vi "SeCrTS-DD Queue Data log module.vi"(8 "error in":errorcluster) -> (0 "error out":errorcluster)   [LabVIEW 2022 SP3]
uses:
  Control/SeCrTS-Datalog enumDD.ctl
  Globals/SeCrTS-DD globals.vi
panel:
  out "x":u32
  out "x-y":dbl
  out "Restart":bool
  out "Log health":bool=TRUE
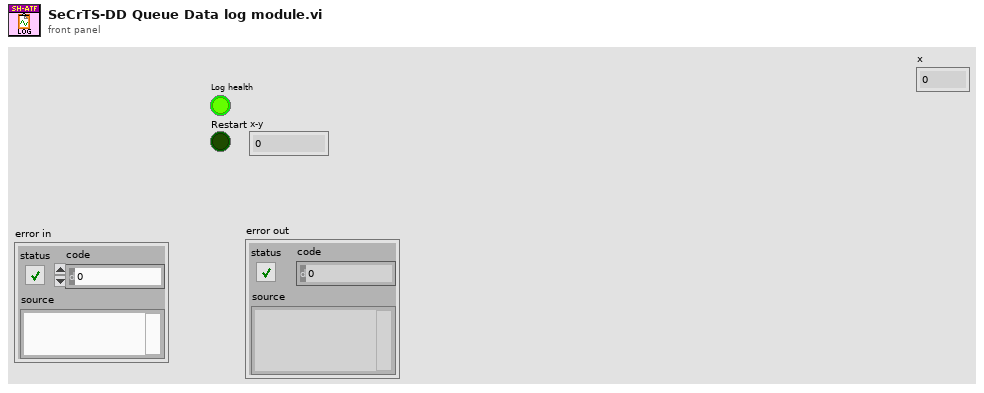
[diagram p1: front panel]
types:
  T1 = cluster{"Log In Progress?":bool, "Log Start Time":timestamp, "Analog Queues":refnum<queue>[], "Digital Queues":refnum<queue>[], "tdms file ref":refnum<k34>}
  T2 = typedef "SeCrTS-Datalog enumDD.ctl" = enum16{"Initialize", "Poll", "Create file", "log Analog", "log Digital", "Flush Queues", "Close file", "Error", "Exit"}
  T3 = enum16{"open", "open or create", "create or replace", "create", "open (read-only)"}
  T4 = cluster{"Datalog path":path, "Configuration path":path, "Signal list path":path, "Sub vi's":path, "Authentication":path}
  T5 = cluster{"Channel names":cluster{"AI_C_Data P":string[], "AI_V_Data P":string[], "AO_Data P":string[], "DO_Data P":string[], "ACC_Data P":string[], "TC Data P":string[], "Drive_A_C":string[], "Drive_A_D":string[], "AI_C_Data S":string[], "DO_Data S":string[]}, "DI Names":cluster{"Di P":string[], "Di S":string[]}}
  T6 = cluster{"AI_C_Data P":string[], "AI_V_Data P":string[], "AO_Data P":string[], "DO_Data P":string[], "ACC_Data P":string[], "TC Data P":string[], "Drive_A_C":string[], "Drive_A_D":string[], "AI_C_Data S":string[], "DO_Data S":string[]}
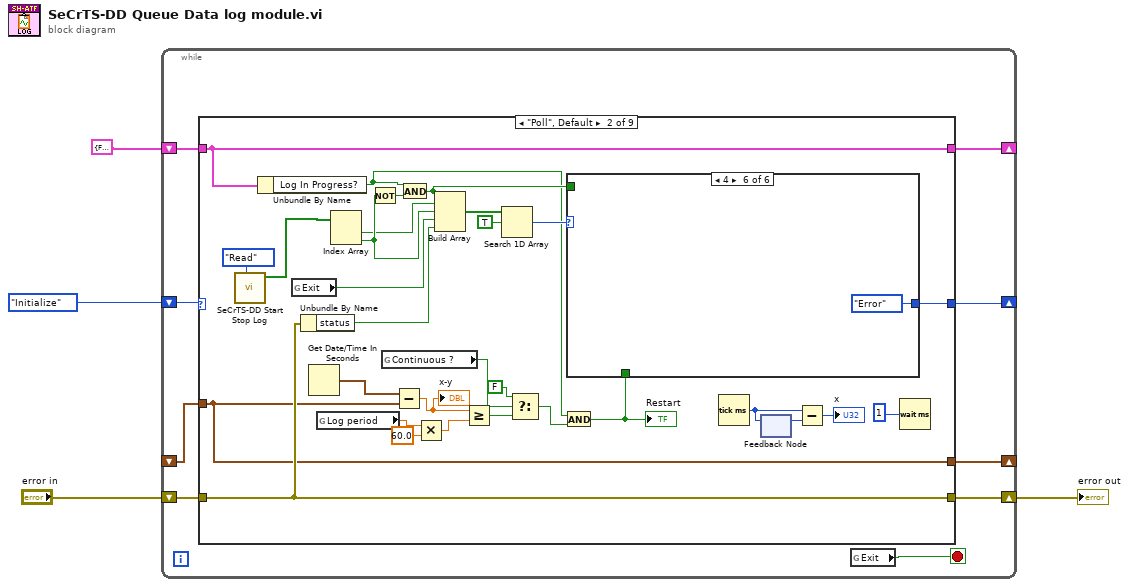
[diagram p0: block diagram]
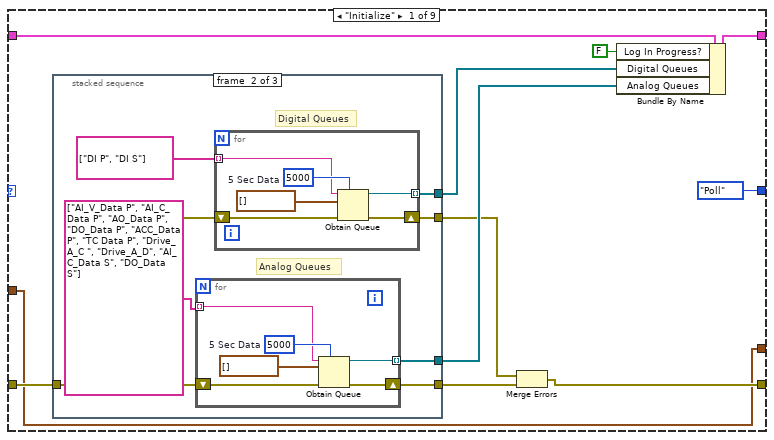
[diagram p2: hidden frame]
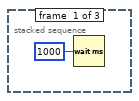
[diagram p3: hidden frame]
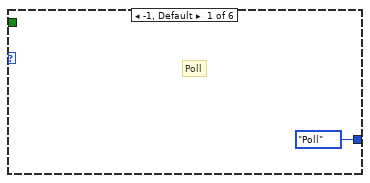
[diagram p5: hidden frame]
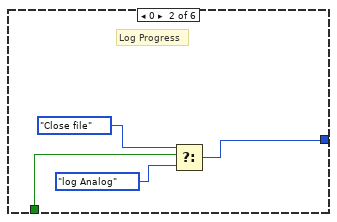
[diagram p6: hidden frame]
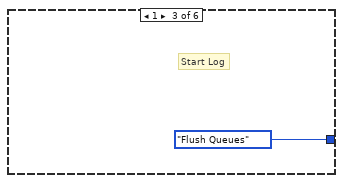
[diagram p7: hidden frame]
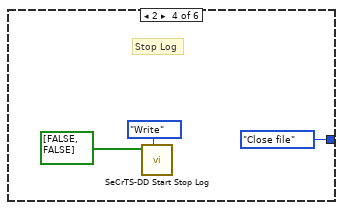
[diagram p8: hidden frame]
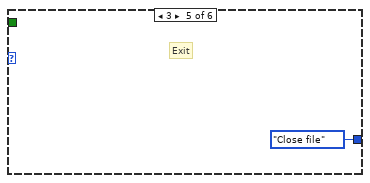
[diagram p9: hidden frame]
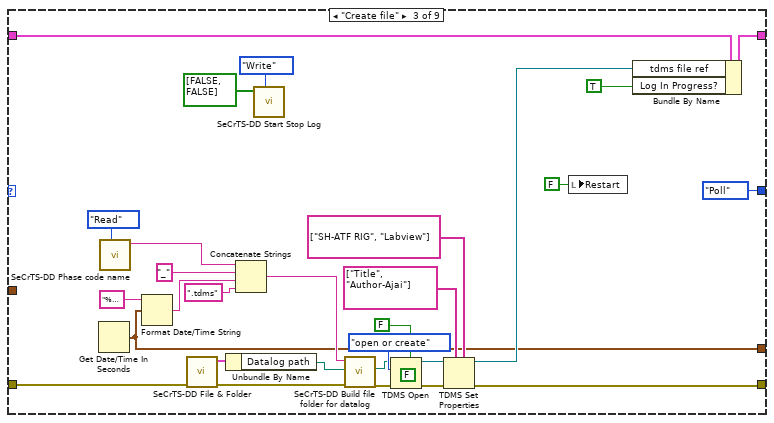
[diagram p10: hidden frame]
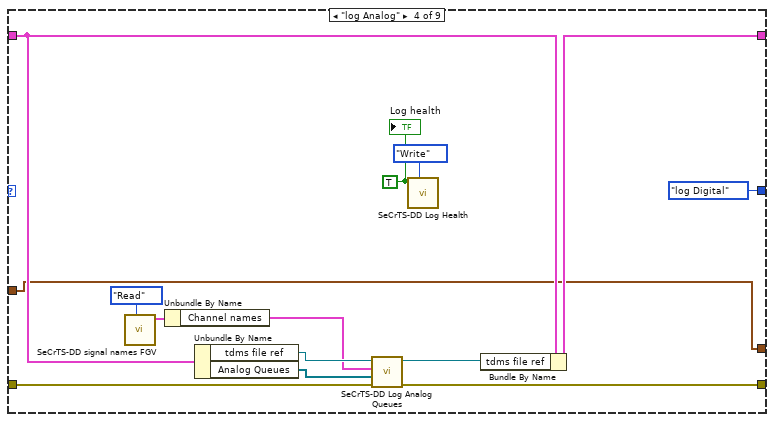
[diagram p11: hidden frame]
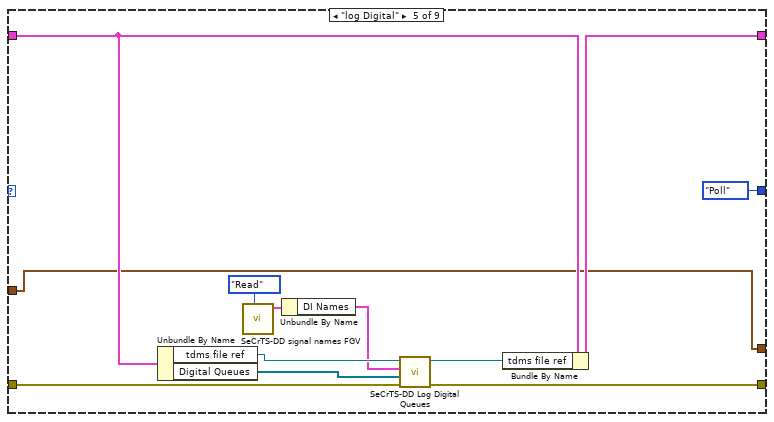
[diagram p12: hidden frame]
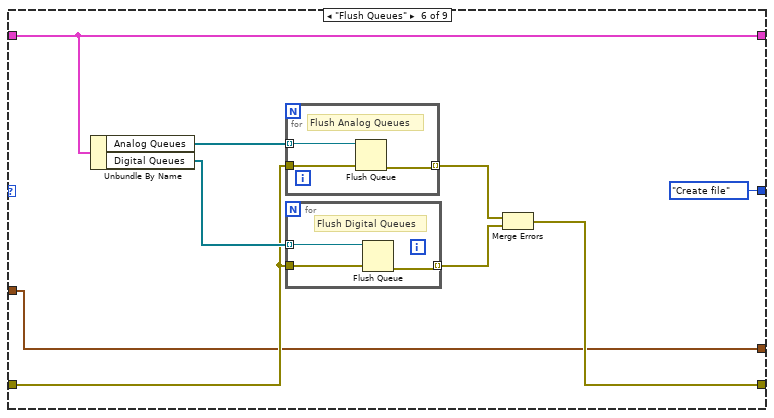
[diagram p13: hidden frame]
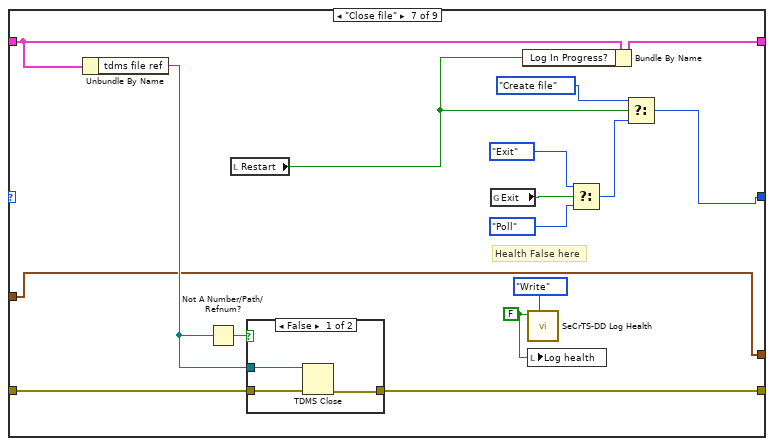
[diagram p14: hidden frame]
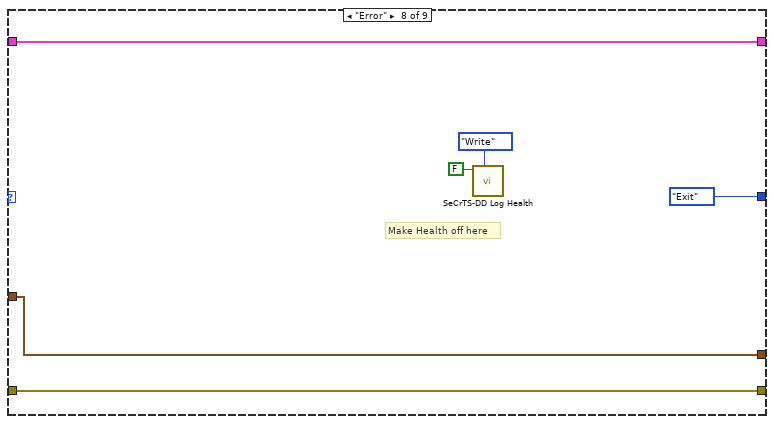
[diagram p16: hidden frame]
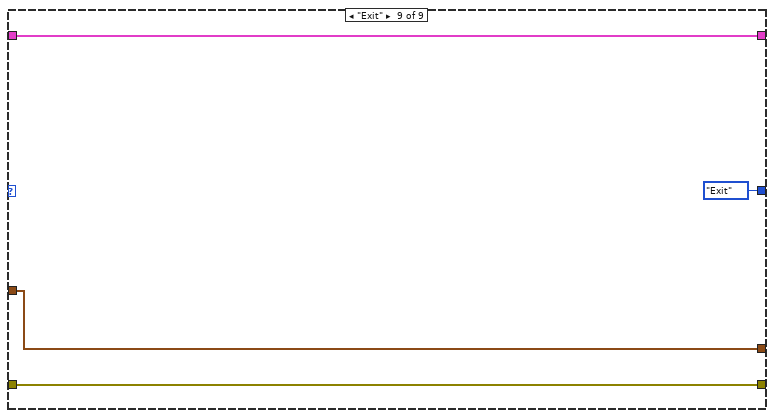
[diagram p17: hidden frame]
diagram:
  n1 = while {
    shift-right: [w8] -> _
    shift-left: SeCrTS-Datalog_enumDD."Initialize" -> [w13]
    shift-right: [w10] -> _
    shift-left: T1 {"Log In Progress?"=FALSE, "Log Start Time"=timestamp(0 s since 1904-01-01), "Analog Queues"=[], "Digital Queues"=[], "tdms file ref"=refnum} -> [w11]
    shift-right: [w9] -> w1
    shift-left: "error in" -> [w12]
    shift-right: [w5] -> _
    shift-left: _ -> [w6]
    stop <- w7 stop-if-true
    n2 = case shown="\"Poll\", Default" w13 {
      tunnel: w12 -> [w23 w68 w109 w125 w139 w145 w167 w179 w184]
      tunnel: w11 -> [w24 w74 w98 w127 w137 w148 w168 w181 w185]
      tunnel: [w22 w74 w97 w122 w134 w148 w169 w181 w185] -> w10
      tunnel: [w16 w68 w94 w124 w138 w142 w166 w179 w184] -> w9
      tunnel: [SeCrTS-Datalog_enumDD."Poll" w69 SeCrTS-Datalog_enumDD."Poll" SeCrTS-Datalog_enumDD."log Digital" SeCrTS-Datalog_enumDD."Poll" SeCrTS-Datalog_enumDD."Create file" w156 SeCrTS-Datalog_enumDD."Exit" SeCrTS-Datalog_enumDD."Exit"] -> w8
      tunnel: w6 -> [w14 w58 _ w115 w129 w141 w160 w176 w182]
      tunnel: [w14 w58 w88 w115 w129 w141 w160 w176 w182] -> w5
      frame "Initialize" {
        n3 = stacked-sequence {
          tunnel: w23 -> [_ w31 _]
          tunnel: [_ w32 _] -> w19
          tunnel: [_ w30 _] -> w20
          tunnel: [_ w29 _] -> w18
          tunnel: [_ w28 _] -> w17
          frame #0 {
            n4 = Wait (ms)(milliseconds to wait=u32 1000) -> ()  [unwired: 1 out]
          }
          frame #1 {
            # "Digital Queues"
            # "Analog Queues"
            n5 = for {
              tunnel: [w41] -> w32 mode=indexing
              shift-right: [w43] -> w28
              shift-left: w31 -> [w44]
              tunnel: string[] ["AI_V_Data P", "AI_C_Data P", "AO_Data P", "DO_Data P", "ACC_Data P", "TC Data P", "Drive_A_C ", "Drive_A_D", "AI_C_Data S", "DO_Data S"] ("Array") -> [w40] mode=indexing
              w42 = 5000  # 5 Sec Data
              n6 = Obtain Queue(max queue size (-1, unlimited)=w42, name (unnamed)=w40, element data type=waveform(dbl)[] [] ("data"), error in (no error)=w44) -> (queue out=w41:refnum<queue>, error out=w43:errorcluster)  [unwired: 1 in, 1 out]
            }
            n7 = for {
              tunnel: [w35] -> w30 mode=indexing
              shift-right: [w37] -> w29
              shift-left: w31 -> [w38]
              tunnel: string[] ["DI P", "DI S"] ("name (unnamed)") -> [w34] mode=indexing
              w36 = 5000  # 5 Sec Data
              n8 = Obtain Queue(max queue size (-1, unlimited)=w36, name (unnamed)=w34, element data type=digitalwaveform[] [] ("data"), error in (no error)=w38) -> (queue out=w35:refnum<queue>, error out=w37:errorcluster)  [unwired: 1 in, 1 out]
            }
          }
          frame #2 {
            # "Datalog loop running Status"
          }
        }
        n9 = Merge Errors(w18, w17) -> (w16:errorcluster)
        n10 = Bundle By Name(cluster=w24, "Log In Progress?"=FALSE, "Digital Queues"=w20, "Analog Queues"=w19) -> (w22:T1)
      }
      frame "Poll", Default {
        n11 = call "SeCrTS-DD Start Stop Log.vi"("Enum"=enum16{"Read", "Write"}."Read") -> ("Start Stop log R"=w54:bool[])  [unwired: 9 in, 1 out]
        n12 = Unbundle By Name(w74) -> ("Log In Progress?"=w48:bool)
        n13 = global read "SeCrTS-DD globals.vi" "Exit"() -> (w64:bool)
        n14 = Unbundle By Name(w68) -> ("status"=w73:bool)
        n15 = Get Date/Time In Seconds() -> (seconds since 1Jan1904=w60:timestamp)
        n16 = global read "SeCrTS-DD globals.vi" "Log period"() -> (w47:dbl)
        n17 = Index Array(array=w54) -> (element #1=w65:bool, element #2=w66:bool)  [unwired: 2 in]
        n18 = Not(x=w66) -> (.not. x?=w67:bool)
        n19 = global read "SeCrTS-DD globals.vi" "Continuous ?"() -> (w52:bool)
        n20 = Subtract(x=w60, y=w58) -> (x-y=w61:dbl)
        "x-y" <- w61
        n21 = And(x=w48, y=w67) -> (x .and. y?=w62:bool)
        n22 = Multiply(x=w47, y=60.0) -> (x*y=w45:dbl)
        n23 = Build Array(w62, w65, w66, w64, w73) -> (w72:bool[])
        n24 = Greater Or Equal?(x=w61, y=w45) -> (x >= y?=w51:bool)
        n25 = Search 1D Array(1D array=w72, element=TRUE) -> (index of element=w70:i32)  [unwired: 1 in]
        n26 = Select(t=FALSE, s=w52, f=w51) -> (s? t:f=w49:bool)
        n27 = And(x=w48, y=w49) -> (x .and. y?=w59:bool)
        "Restart" <- w59
        n28 = case shown="4" w70 {
          tunnel: [SeCrTS-Datalog_enumDD."Poll" w76 SeCrTS-Datalog_enumDD."Flush Queues" SeCrTS-Datalog_enumDD."Close file" SeCrTS-Datalog_enumDD."Close file" SeCrTS-Datalog_enumDD."Error"] -> w69
          tunnel: w62 -> [_ _ _ _ _ _]
          tunnel: w59 -> [_ w79 _ _ _ _]
          frame -1, Default {
            # "Poll"
          }
          frame 0 {
            # "Log Progress"
            n29 = Select(t=SeCrTS-Datalog_enumDD."Close file", s=w79, f=SeCrTS-Datalog_enumDD."log Analog") -> (s? t:f=w76:T2)
          }
          frame 1 {
            # "Start Log"
          }
          frame 2 {
            # "Stop Log"
            n30 = call "SeCrTS-DD Start Stop Log.vi"("Enum"=enum16{"Read", "Write"}."Write", "Start Stop log"=bool[] [FALSE, FALSE]) -> ()  [unwired: 8 in, 2 out]
          }
          frame 3 {
            # "Exit"
          }
          frame 4 {
          }
        }
        n31 = Tick Count (ms)() -> (millisecond timer value=w56:u32)
        n32 = feedback #1() -> (w57:u32)  [unwired: 1 in]
        n33 = feedback-in #1(w56) -> ()
        n34 = Subtract(x=w56, y=w57) -> (x-y=→"x":u32)
        n35 = Wait (ms)(milliseconds to wait=u32 1 ("millisecond timer value")) -> ()  [unwired: 1 out]
      }
      frame "Create file" {
        (unwired) FALSE ("disable buffering? (T)")
        n36 = Get Date/Time In Seconds() -> (seconds since 1Jan1904=w88:timestamp)
        n37 = call "SeCrTS-DD Phase code name.vi"("Enum"=enum16{"Read", "Write"}."Read") -> ("Phase codeR"=w89:string)  [unwired: 9 in, 1 out]
        n38 = Format Date/Time String(time format string (%c)="%Y_%b_%d_%Hh_%Mm_%Ssec", seconds (now)=w88) -> (date/time string=w114:string)  [unwired: 1 in]
        n39 = call "SeCrTS-DD File & Folder.vi"("error in (no error)"=w109) -> ("error out"=w108:errorcluster, "File Output"=w107:T4)  [unwired: 9 in]
        n40 = Unbundle By Name(w107) -> ("Datalog path"=w106:path)
        n41 = Concatenate Strings(w89, "_" ("string"), w114, ".tdms" ("string")) -> (w110:string)
        n42 = call "SeCrTS-DD Start Stop Log.vi"("Enum"=enum16{"Read", "Write"}."Write", "Start Stop log"=bool[] [FALSE, FALSE]) -> ()  [unwired: 8 in, 2 out]
        n43 = call "SeCrTS-DD Build file folder for datalog.vi"("error in (no error)"=w108, "Base Path"=w106, "File Name"=w110) -> ("error out"=w100:errorcluster, "Result File path"=w99:path)  [unwired: 6 in, 1 out]
        n44 = TDMS Open(5:FALSE ("create index file? (T)"), 8:w100, 10:T3."open or create" ("operation (0:open)"), 11:w99) -> (0:w104:errorcluster, 3:w103:refnum<k34>)  [unwired: 3 in]
        n45 = TDMS Set Properties(5:string[] ["SH-ATF RIG", "Labview"] ("property names"), 7:string[] ["Title", "Author-Ajai"] ("property names"), 8:w104, 11:w103) -> (0:w94:errorcluster, 3:w96:refnum<k34>)  [unwired: 4 out]
        n46 = local write "Restart"(FALSE ("Restart")) -> ()
        n47 = Bundle By Name(cluster=w98, "tdms file ref"=w96, "Log In Progress?"=TRUE) -> (w97:T1)
      }
      frame "log Analog" {
        w119 = TRUE ("Log health")
        n48 = call "SeCrTS-DD signal names FGV.vi"("Enum"=enum16{"Read", "Write"}."Read") -> ("Signal names"=w117:T5)  [unwired: 9 in, 1 out]
        n49 = Unbundle By Name(w117) -> ("Channel names"=w116:T6)
        n50 = Unbundle By Name(w127) -> ("tdms file ref"=w123:refnum<k34>, "Analog Queues"=w126:refnum<queue>[])
        n51 = call "SeCrTS-DD Log Analog Queues.vi"("error in"=w125, "Analog queues"=w126, "Channel names"=w116, "tdms file in"=w123) -> ("error out"=w124:errorcluster, "tdms ref out"=w121:refnum<k34>)  [unwired: 6 in]
        n52 = call "SeCrTS-DD Log Health.vi"("Enum"=enum16{"Read", "Write"}."Write", "Log health"=w119) -> ()  [unwired: 8 in, 2 out]
        n53 = Bundle By Name(cluster=w127, "tdms file ref"=w121) -> (w122:T1)
        "Log health" <- w119
      }
      frame "log Digital" {
        n54 = Unbundle By Name(w137) -> ("tdms file ref"=w136:refnum<k34>, "Digital Queues"=w135:refnum<queue>[])
        n55 = call "SeCrTS-DD signal names FGV.vi"("Enum"=enum16{"Read", "Write"}."Read") -> ("Signal names"=w131:T5)  [unwired: 9 in, 1 out]
        n56 = Unbundle By Name(w131) -> ("DI Names"=w130:cluster{"Di P":string[], "Di S":string[]})
        n57 = call "SeCrTS-DD Log Digital Queues.vi"("error in"=w139, "DI_queue"=w135, "DI Names 2"=w130, "tdms file in"=w136) -> ("error out"=w138:errorcluster, "tdms file out"=w133:refnum<k34>)  [unwired: 6 in]
        n58 = Bundle By Name(cluster=w137, "tdms file ref"=w133) -> (w134:T1)
      }
      frame "Flush Queues" {
        n59 = Unbundle By Name(w148) -> ("Analog Queues"=w147:refnum<queue>[], "Digital Queues"=w146:refnum<queue>[])
        n60 = for {
          tunnel: w147 -> [w155] mode=indexing
          tunnel: w145 -> [w154]
          tunnel: [w153] -> w144 mode=indexing
          # "Flush Analog Queues"
          n61 = Flush Queue(queue=w155, error in (no error)=w154) -> (error out=w153:errorcluster)  [unwired: 2 out]
        }
        n62 = for {
          tunnel: w146 -> [w152] mode=indexing
          tunnel: w145 -> [w151]
          tunnel: [w150] -> w143 mode=indexing
          # "Flush Digital Queues"
          n63 = Flush Queue(queue=w152, error in (no error)=w151) -> (error out=w150:errorcluster)  [unwired: 2 out]
        }
        n64 = Merge Errors(w144, w143) -> (w142:errorcluster)
      }
      frame "Close file" {
        w161 = FALSE ("Log health")
        # "Health False here"
        n65 = Unbundle By Name(w168) -> ("tdms file ref"=w164:refnum<k34>)
        n66 = Not A Number/Path/Refnum?(number/path/refnum=w164) -> (NaN/Path/Refnum?=w165:bool)
        n67 = local read "Restart"() -> (w159:bool)
        n68 = case shown="False" w165 {
          tunnel: w167 -> [w174 w175]
          tunnel: [w173 w175] -> w166
          tunnel: w164 -> [w172 _]
          frame False {
            n69 = TDMS Close(8:w174, 11:w172) -> (0:w173:errorcluster)  [unwired: 1 out]
          }
          frame True {
          }
        }
        n70 = global read "SeCrTS-DD globals.vi" "Exit"() -> (w162:bool)
        n71 = Bundle By Name(cluster=w168, "Log In Progress?"=w159) -> (w169:T1)
        n72 = call "SeCrTS-DD Log Health.vi"("Enum"=enum16{"Read", "Write"}."Write", "Log health"=w161) -> ()  [unwired: 8 in, 2 out]
        n73 = local write "Log health"(w161) -> ()
        n74 = Select(t=SeCrTS-Datalog_enumDD."Exit", s=w162, f=SeCrTS-Datalog_enumDD."Poll") -> (s? t:f=w157:T2)
        n75 = Select(t=SeCrTS-Datalog_enumDD."Create file", s=w159, f=w157) -> (s? t:f=w156:T2)
      }
      frame "Error" {
        # "Make Health off here"
        n76 = call "SeCrTS-DD Log Health.vi"("Enum"=enum16{"Read", "Write"}."Write", "Log health"=FALSE) -> ()  [unwired: 8 in, 2 out]
      }
      frame "Exit" {
      }
    }
    n77 = global read "SeCrTS-DD globals.vi" "Exit"() -> (w7:bool)
  }
  "error out" <- w1
